vi "Set Output Values.vi"(8 "error in (no error)":errorcluster, 11 "Spectrum Recorder in":refnum<class "Spectrum Recorder too.lvclass">) -> (0 "error out":errorcluster, 3 "Spectrum Recorder out":refnum<class "Spectrum Recorder too.lvclass">)   [LabVIEW 2016, in "Spectrum Recorder too.lvclass"]
uses:
  Spectrum Recorder too.lvclass
  Spectrum Recorder too.lvclass/Spectrum Recorder too.ctl
  Read Spectrum Recorder Configuration.vi
  Read RP transceiver.vi
  Write RP transceiver.vi
  NHMFL_Core/Libraries/Red Pitaya/RP Core/RP Transceiver/RP Transceiver.lvclass
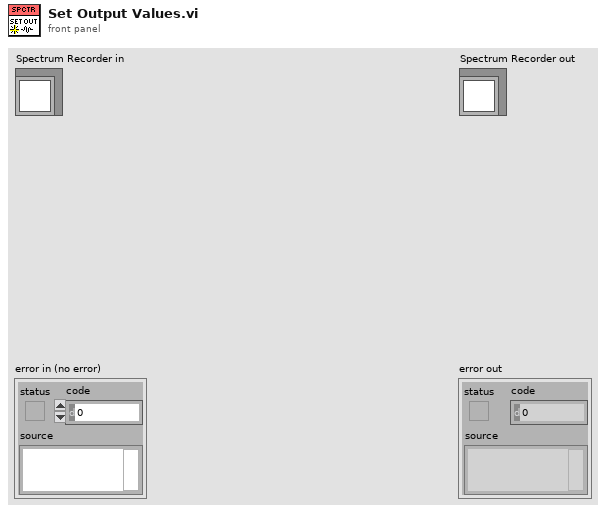
[diagram p1: front panel]
types:
  T1 = typedef "Spectrum Configuration.ctl" = cluster{"Start frequency":dbl, "End frequency":dbl, "Coarse step":dbl, "Step duration":dbl, "Red Pitaya address":string, "Open plot \non start":bool, "Fine region centers":dbl[], "Regions width":dbl, "Fine step":dbl, "Pause between scans":dbl, "Clear rgs on start":bool}
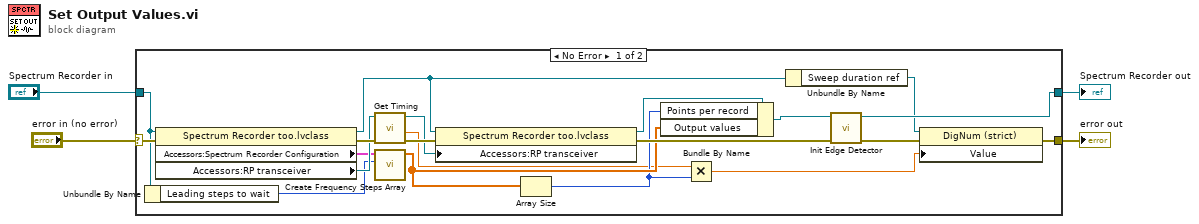
[diagram p0: block diagram]
diagram:
  n1 = case shown="No Error" "error in (no error)" {
    selector: "error in (no error)" -> [w21 w26]
    tunnel: [w11 w26] -> w3
    tunnel: [w16 w25] -> w1
    tunnel: "Spectrum Recorder in" -> [w6 w25]
    frame No Error {
      n2 = Unbundle By Name(w6) -> ("Leading steps to wait"=w5:i32)
      n3 = property class="Spectrum Recorder too.lvclass"(reference=w6, error in=w21) -> (reference out=w14:refnum<class "Spectrum Recorder too.lvclass">, error out=w22:errorcluster, "Accessors:Spectrum Recorder Configuration"=w7:T1, "Accessors:RP transceiver"=w20:refnum<class "RP Transceiver.lvclass">)
      n4 = call-dynamic "Get Timing.vi"("error in (no error)"=w22, "RP Transceiver in"=w20) -> ("error out"=w24:errorcluster, "dt"=w9:dbl, "RP Transceiver out"=w23:refnum<class "RP Transceiver.lvclass">)  [unwired: 5 in, 2 out]
      n5 = call "Create Frequency Steps Array.vi"("Leading steps to wait"=w5, "Spectrum Recorder Configuration"=w7) -> ("Steps"=w15:dbl[])  [unwired: 9 in]
      n6 = property class="Spectrum Recorder too.lvclass"(reference=w14, error in=w24, "Accessors:RP transceiver"=w23) -> (reference out=w19:refnum<class "Spectrum Recorder too.lvclass">, error out=w17:errorcluster)
      n7 = Array Size(array=w15) -> (size(s)=w10:i32)
      n8 = Bundle By Name(cluster=w19, "Points per record"=w10, "Output values"=w15) -> (w18:refnum<class "Spectrum Recorder too.lvclass">)
      n9 = Multiply(x=w9, y=w10) -> (x*y=w8:dbl)
      n10 = Unbundle By Name(w14) -> ("Sweep duration ref"=w13:refnum<vi>)
      n11 = call-dynamic "Init Edge Detector.vi"("error in (no error)"=w17, "Spectrum Recorder too in"=w18) -> ("error out"=w12:errorcluster, "Spectrum Recorder too out"=w16:refnum<class "Spectrum Recorder too.lvclass">)  [unwired: 8 in]
      n12 = property class="DigNum (strict)"(reference=w13, error in=w12, "Value"=w8) -> (error out=w11:errorcluster)  [unwired: 1 out]
    }
    frame Error {
    }
  }
  "error out" <- w3
  "Spectrum Recorder out" <- w1
